vi "cmd_vel.vi"(10 "Angular.z":dbl, 11 "Linear.x":dbl) -> (3 "msg out":string)   [LabVIEW 2014]
uses:
  ctl/twist.ctl
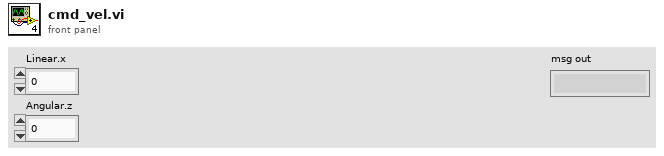
[diagram p1: front panel]
types:
  T1 = typedef "twist.ctl" = cluster{"Linear":cluster{"x":dbl, "y":dbl, "z":dbl}, "Angular":cluster{"x":dbl, "y":dbl, "z":dbl}}
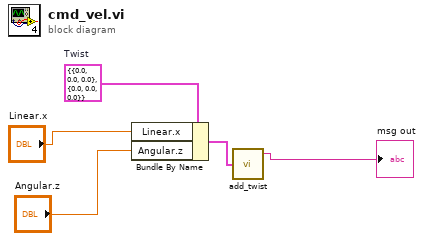
[diagram p0: block diagram]
diagram:
  w5 = T1 {"Linear"={"x"=0.0, "y"=0.0, "z"=0.0}, "Angular"={"x"=0.0, "y"=0.0, "z"=0.0}}  # Twist
  n1 = Bundle By Name(cluster=w5, "Linear.x"="Linear.x", "Angular.z"="Angular.z") -> (w4:T1)
  n2 = call <vilib>:"add_twist.vi"("Twist"=w4) -> ("msg out"=→"msg out":string)  [unwired: 4 in]
